vi "CalculateTorque.vi"(4 "Frequency":dbl, 5 "TranslationPosition":dbl, 6 "Sensors Right":T1, 7 "Sensors Left":T1) -> (3 "Torque":dbl)   [LabVIEW 2019]
uses:
  <vilib>/Utility/miscctls.llb/LV3DPointTypeDef.ctl
  <vilib>/Analysis/Matrix/Datatypes/RealMatrix.ctl
  TypeDefs/SensorControl.ctl
  <vilib>/Analysis/3filter.llb/Filter Passband Type.ctl
  <vilib>/Analysis/_algsub.llb/Real Vector Norm.vi
  <vilib>/Analysis/baseanly.llb/A x Vector.vi
  <vilib>/Analysis/NI_AALBase.lvlib
  <vilib>/Analysis/NI_AALPro.lvlib
  <vilib>/ptbypt/NI_PtbyPt.lvlib
  <vilib>/Analysis/Matrix/NI_Matrix.lvlib
panel:
  out "RotMatrix":T2
  out "size right":i32
  out "Vertex Array right":T3[](array[typedef])
  out "triangle":dbl[](array[numeric])
  out "size left":i32
  out "Vertex Array left":T3[](array[typedef])
  out "Low Cutoff":dbl=30.0
  out "t_right":dbl format="%.2f"
  out "intersect_right":bool
  out "t_left":dbl format="%.2f"
  out "intersect_left":bool
  out "dir left":dbl[](array[numeric])
  out "orig left":dbl[](array[numeric])
  out "dir right":dbl[](array[numeric])
  out "orig right":dbl[](array[numeric])
  out "force left":dbl[](array[numeric])
  out "force right":dbl[](array[numeric])
  out "torque left":dbl[](array[numeric])
  out "torque right":dbl[](array[numeric])
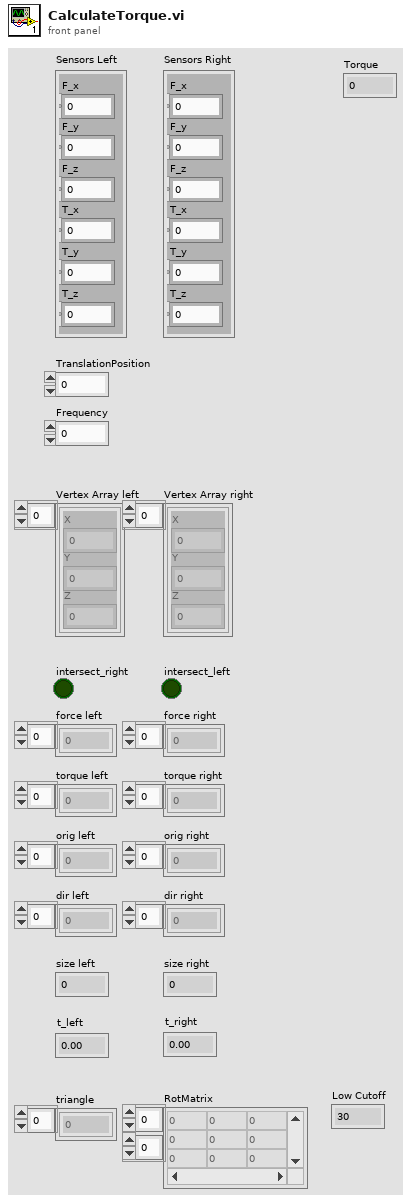
[diagram p1: front panel]
types:
  T1 = typedef "SensorControl.ctl" = cluster{"F_x":dbl, "F_y":dbl, "F_z":dbl, "T_x":dbl, "T_y":dbl, "T_z":dbl}
  T2 = typedef "NI_Matrix.lvlib/RealMatrix.ctl" = dbl[][]
  T3 = typedef "LV3DPointTypeDef.ctl" = cluster{"X":sgl, "Y":sgl, "Z":sgl}
  T4 = typedef "NI_AALBase.lvlib/Filter Passband Type.ctl" = enum32{"Lowpass", "Highpass", "Bandpass", "Bandstop"}
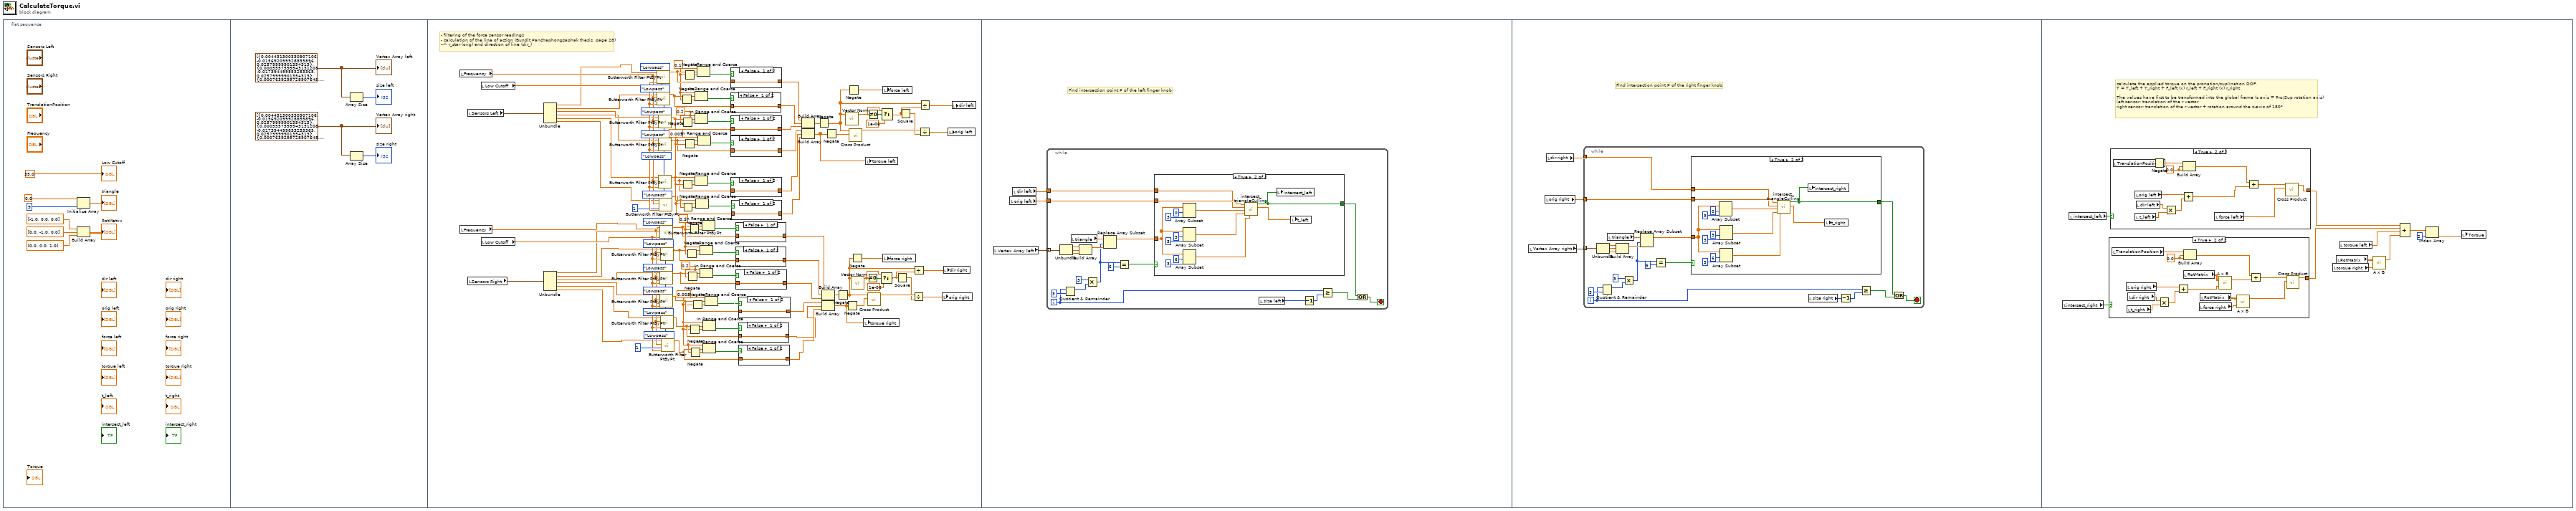
[diagram p0: block diagram]
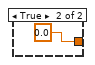
[diagram p2: hidden frame]
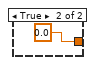
[diagram p3: hidden frame]
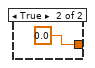
[diagram p4: hidden frame]
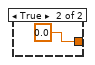
[diagram p5: hidden frame]
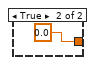
[diagram p6: hidden frame]
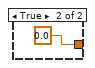
[diagram p7: hidden frame]
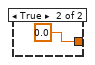
[diagram p8: hidden frame]
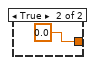
[diagram p9: hidden frame]
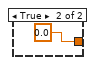
[diagram p10: hidden frame]
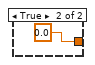
[diagram p11: hidden frame]
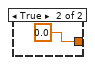
[diagram p12: hidden frame]
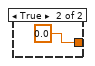
[diagram p13: hidden frame]
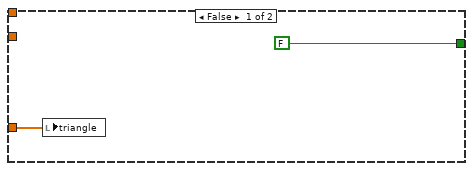
[diagram p14: hidden frame]
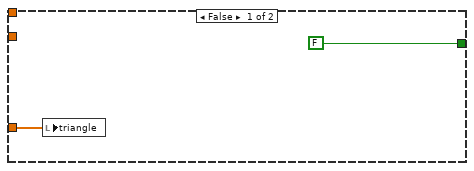
[diagram p15: hidden frame]
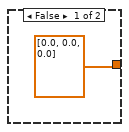
[diagram p16: hidden frame]
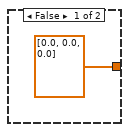
[diagram p17: hidden frame]
diagram:
  n1 = flat-sequence {
    frame #0 {
      n2 = Initialize Array(0.0 ("element"), 9 ("dimension size")) -> (→"triangle":dbl[])
      n3 = Build Array(dbl[] [-1.0, 0.0, 0.0] ("element"), dbl[] [0.0, -1.0, 0.0] ("element"), dbl[] [0.0, 0.0, 1.0] ("element")) -> (→"RotMatrix":T2)
      "Low Cutoff" <- 35.0
    }
    frame #1 {
      w11 = T3[] [{"X"=0.0044313003, "Y"=-0.0156921, "Z"=0.025799999}, {"X"=0.00055576, "Y"=-0.0173945, "Z"=0.025799999}, {"X"=0.00076393, "Y"=-0.02, "Z"=0.025799999}, {"X"=0.00076393, "Y"=-0.02, "Z"=0.025799999}, {"X"=0.00076393, "Y"=-0.02, "Z"=0.0088}, {"X"=0.00055576, "Y"=-0.0173945, "Z"=0.0088}, {"X"=0.00044313, "Y"=-0.0156921, "Z"=0.025799999}, {"X"=0.00055576, "Y"=-0.0173945, "Z"=0.0088}, {"X"=0.00044313, "Y"=-0.0156921, "Z"=0.0088}, {"X"=0.00044313, "Y"=-0.0156921, "Z"=0.025799999}, {"X"=0.00076393, "Y"=-0.02, "Z"=0.025799999}, {"X"=0.00055576, "Y"=-0.0173945, "Z"=0.0088}, {"X"=0.00044313, "Y"=-0.0156921, "Z"=0.0088}, {"X"=0.0002803, "Y"=-0.012661899, "Z"=0.0088}, {"X"=0.0002803, "Y"=-0.012661899, "Z"=0.025799999}, {"X"=0.0002803, "Y"=-0.012661899, "Z"=0.025799999}, {"X"=0.00044313, "Y"=-0.0156921, "Z"=0.025799999}, {"X"=0.00044313, "Y"=-0.0156921, "Z"=0.0088}, {"X"=0.00026629, "Y"=-0.0120288, "Z"=0.025799999}, {"X"=0.00026629, "Y"=-0.0120288, "Z"=0.0088}, {"X"=0.00028451, "Y"=-0.0113124, "Z"=0.0088}, {"X"=0.00030813, "Y"=-0.0109895, "Z"=0.0088}, {"X"=0.00033954, "Y"=-0.01074, "Z"=0.0088}, {"X"=0.00033954, "Y"=-0.01074, "Z"=0.025799999}, {"X"=0.00033954, "Y"=-0.01074, "Z"=0.025799999}, {"X"=0.00026629, "Y"=-0.0120288, "Z"=0.025799999}, {"X"=0.00028451, "Y"=-0.0113124, "Z"=0.0088}, {"X"=0.00028451, "Y"=-0.0113124, "Z"=0.0088}, {"X"=0.00030813, "Y"=-0.0109895, "Z"=0.0088}, {"X"=0.00033954, "Y"=-0.01074, "Z"=0.025799999}, {"X"=0.00026629, "Y"=-0.0120288, "Z"=0.0088}, {"X"=0.00026629, "Y"=-0.0120288, "Z"=0.025799999}, {"X"=0.0002803, "Y"=-0.012661899, "Z"=0.025799999}, {"X"=0.0002803, "Y"=-0.012661899, "Z"=0.025799999}, {"X"=0.0002803, "Y"=-0.012661899, "Z"=0.0088}, {"X"=0.00026629, "Y"=-0.0120288, "Z"=0.0088}, {"X"=0.00044204, "Y"=-0.0100592, "Z"=0.025799999}, {"X"=0.00033954, "Y"=-0.01074, "Z"=0.025799999}, {"X"=0.00033954, "Y"=-0.01074, "Z"=0.0088}, {"X"=0.00033954, "Y"=-0.01074, "Z"=0.0088}, {"X"=0.00079033, "Y"=-0.0061129997, "Z"=0.0088}, {"X"=0.00079033, "Y"=-0.0061129997, "Z"=0.025799999}, {"X"=0.00079033, "Y"=-0.0061129997, "Z"=0.025799999}, {"X"=0.00044204, "Y"=-0.0100592, "Z"=0.025799999}, {"X"=0.00033954, "Y"=-0.01074, "Z"=0.0088}, {"X"=0.00094135, "Y"=-0.0014677, "Z"=0.025799999}, {"X"=0.00079033, "Y"=-0.0061129997, "Z"=0.025799999}, {"X"=0.00079033, "Y"=-0.0061129997, "Z"=0.0088}, {"X"=0.00079033, "Y"=-0.0061129997, "Z"=0.0088}, {"X"=0.00095, "Y"=0.0, "Z"=0.0088}, {"X"=0.00095, "Y"=0.0, "Z"=0.025799999}, {"X"=0.00095, "Y"=0.0, "Z"=0.025799999}, {"X"=0.00094135, "Y"=-0.0014677, "Z"=0.025799999}, {"X"=0.00079033, "Y"=-0.0061129997, "Z"=0.0088}, {"X"=0.00079033, "Y"=0.0061129997, "Z"=0.025799999}, {"X"=0.00095, "Y"=0.0, "Z"=0.025799999}, {"X"=0.00095, "Y"=0.0, "Z"=0.0088}, {"X"=0.00095, "Y"=0.0, "Z"=0.0088}, {"X"=0.00079033, "Y"=0.0061129997, "Z"=0.0088}, {"X"=0.00079033, "Y"=0.0061129997, "Z"=0.025799999}, {"X"=0.00079033, "Y"=0.0061129997, "Z"=0.0088}, {"X"=0.00053803, "Y"=0.0092747, "Z"=0.0088}, {"X"=0.00033954, "Y"=0.01074, "Z"=0.0088}, {"X"=0.00033954, "Y"=0.01074, "Z"=0.0088}, {"X"=0.00033954, "Y"=0.01074, "Z"=0.025799999}, {"X"=0.00067254, "Y"=0.007852701, "Z"=0.025799999}, {"X"=0.00067254, "Y"=0.007852701, "Z"=0.025799999}, {"X"=0.00079033, "Y"=0.0061129997, "Z"=0.025799999}, {"X"=0.00079033, "Y"=0.0061129997, "Z"=0.0088}, {"X"=0.00079033, "Y"=0.0061129997, "Z"=0.0088}, {"X"=0.00033954, "Y"=0.01074, "Z"=0.0088}, {"X"=0.00067254, "Y"=0.007852701, "Z"=0.025799999}, {"X"=0.00026629, "Y"=0.0120289, "Z"=0.025799999}, {"X"=0.00026629, "Y"=0.0120289, "Z"=0.0088}, {"X"=0.0002803, "Y"=0.012661899, "Z"=0.0088}, {"X"=0.0002803, "Y"=0.012661899, "Z"=0.0088}, {"X"=0.0002803, "Y"=0.012661899, "Z"=0.025799999}, {"X"=0.00026629, "Y"=0.0120289, "Z"=0.025799999}, {"X"=0.00026629, "Y"=0.0120289, "Z"=0.0088}, {"X"=0.00026629, "Y"=0.0120289, "Z"=0.025799999}, {"X"=0.0002845, "Y"=0.0113124, "Z"=0.025799999}, {"X"=0.00030813, "Y"=0.0109895, "Z"=0.025799999}, {"X"=0.00033954, "Y"=0.01074, "Z"=0.025799999}, {"X"=0.00033954, "Y"=0.01074, "Z"=0.0088}, {"X"=0.00033954, "Y"=0.01074, "Z"=0.0088}, {"X"=0.00026629, "Y"=0.0120289, "Z"=0.0088}, {"X"=0.0002845, "Y"=0.0113124, "Z"=0.025799999}, {"X"=0.0002845, "Y"=0.0113124, "Z"=0.025799999}, {"X"=0.00030813, "Y"=0.0109895, "Z"=0.025799999}, {"X"=0.00033954, "Y"=0.01074, "Z"=0.0088}, {"X"=0.00044313, "Y"=0.0156921, "Z"=0.025799999}, {"X"=0.0002803, "Y"=0.012661899, "Z"=0.025799999}, {"X"=0.0002803, "Y"=0.012661899, "Z"=0.0088}, {"X"=0.0002803, "Y"=0.012661899, "Z"=0.0088}, {"X"=0.00044313, "Y"=0.0156921, "Z"=0.0088}, {"X"=0.00044313, "Y"=0.0156921, "Z"=0.025799999}, {"X"=0.00062176, "Y"=0.0182866, "Z"=0.0088}, {"X"=0.00076393, "Y"=0.02, "Z"=0.0088}, {"X"=0.00076393, "Y"=0.02, "Z"=0.025799999}, {"X"=0.00055576, "Y"=0.0173945, "Z"=0.025799999}, {"X"=0.00044313, "Y"=0.0156921, "Z"=0.025799999}, {"X"=0.00044313, "Y"=0.0156921, "Z"=0.0088}, {"X"=0.00044313, "Y"=0.0156921, "Z"=0.0088}, {"X"=0.00062176, "Y"=0.0182866, "Z"=0.0088}, {"X"=0.00076393, "Y"=0.02, "Z"=0.025799999}, {"X"=0.00076393, "Y"=0.02, "Z"=0.025799999}, {"X"=0.00055576, "Y"=0.0173945, "Z"=0.025799999}, {"X"=0.00044313, "Y"=0.0156921, "Z"=0.0088}] ("Vertex Array left")
      w10 = T3[] [{"X"=0.0044313003, "Y"=-0.0156921, "Z"=0.025799999}, {"X"=0.00055576, "Y"=-0.0173945, "Z"=0.025799999}, {"X"=0.00076393, "Y"=-0.02, "Z"=0.025799999}, {"X"=0.00076393, "Y"=-0.02, "Z"=0.025799999}, {"X"=0.00076393, "Y"=-0.02, "Z"=0.0088}, {"X"=0.00055576, "Y"=-0.0173945, "Z"=0.0088}, {"X"=0.00044313, "Y"=-0.0156921, "Z"=0.025799999}, {"X"=0.00055576, "Y"=-0.0173945, "Z"=0.0088}, {"X"=0.00044313, "Y"=-0.0156921, "Z"=0.0088}, {"X"=0.00044313, "Y"=-0.0156921, "Z"=0.025799999}, {"X"=0.00076393, "Y"=-0.02, "Z"=0.025799999}, {"X"=0.00055576, "Y"=-0.0173945, "Z"=0.0088}, {"X"=0.00044313, "Y"=-0.0156921, "Z"=0.0088}, {"X"=0.0002803, "Y"=-0.012661899, "Z"=0.0088}, {"X"=0.0002803, "Y"=-0.012661899, "Z"=0.025799999}, {"X"=0.0002803, "Y"=-0.012661899, "Z"=0.025799999}, {"X"=0.00044313, "Y"=-0.0156921, "Z"=0.025799999}, {"X"=0.00044313, "Y"=-0.0156921, "Z"=0.0088}, {"X"=0.00026629, "Y"=-0.0120288, "Z"=0.025799999}, {"X"=0.00026629, "Y"=-0.0120288, "Z"=0.0088}, {"X"=0.00028451, "Y"=-0.0113124, "Z"=0.0088}, {"X"=0.00030813, "Y"=-0.0109895, "Z"=0.0088}, {"X"=0.00033954, "Y"=-0.01074, "Z"=0.0088}, {"X"=0.00033954, "Y"=-0.01074, "Z"=0.025799999}, {"X"=0.00033954, "Y"=-0.01074, "Z"=0.025799999}, {"X"=0.00026629, "Y"=-0.0120288, "Z"=0.025799999}, {"X"=0.00028451, "Y"=-0.0113124, "Z"=0.0088}, {"X"=0.00028451, "Y"=-0.0113124, "Z"=0.0088}, {"X"=0.00030813, "Y"=-0.0109895, "Z"=0.0088}, {"X"=0.00033954, "Y"=-0.01074, "Z"=0.025799999}, {"X"=0.00026629, "Y"=-0.0120288, "Z"=0.0088}, {"X"=0.00026629, "Y"=-0.0120288, "Z"=0.025799999}, {"X"=0.0002803, "Y"=-0.012661899, "Z"=0.025799999}, {"X"=0.0002803, "Y"=-0.012661899, "Z"=0.025799999}, {"X"=0.0002803, "Y"=-0.012661899, "Z"=0.0088}, {"X"=0.00026629, "Y"=-0.0120288, "Z"=0.0088}, {"X"=0.00044204, "Y"=-0.0100592, "Z"=0.025799999}, {"X"=0.00033954, "Y"=-0.01074, "Z"=0.025799999}, {"X"=0.00033954, "Y"=-0.01074, "Z"=0.0088}, {"X"=0.00033954, "Y"=-0.01074, "Z"=0.0088}, {"X"=0.00079033, "Y"=-0.0061129997, "Z"=0.0088}, {"X"=0.00079033, "Y"=-0.0061129997, "Z"=0.025799999}, {"X"=0.00079033, "Y"=-0.0061129997, "Z"=0.025799999}, {"X"=0.00044204, "Y"=-0.0100592, "Z"=0.025799999}, {"X"=0.00033954, "Y"=-0.01074, "Z"=0.0088}, {"X"=0.00094135, "Y"=-0.0014677, "Z"=0.025799999}, {"X"=0.00079033, "Y"=-0.0061129997, "Z"=0.025799999}, {"X"=0.00079033, "Y"=-0.0061129997, "Z"=0.0088}, {"X"=0.00079033, "Y"=-0.0061129997, "Z"=0.0088}, {"X"=0.00095, "Y"=0.0, "Z"=0.0088}, {"X"=0.00095, "Y"=0.0, "Z"=0.025799999}, {"X"=0.00095, "Y"=0.0, "Z"=0.025799999}, {"X"=0.00094135, "Y"=-0.0014677, "Z"=0.025799999}, {"X"=0.00079033, "Y"=-0.0061129997, "Z"=0.0088}, {"X"=0.00079033, "Y"=0.0061129997, "Z"=0.025799999}, {"X"=0.00095, "Y"=0.0, "Z"=0.025799999}, {"X"=0.00095, "Y"=0.0, "Z"=0.0088}, {"X"=0.00095, "Y"=0.0, "Z"=0.0088}, {"X"=0.00079033, "Y"=0.0061129997, "Z"=0.0088}, {"X"=0.00079033, "Y"=0.0061129997, "Z"=0.025799999}, {"X"=0.00079033, "Y"=0.0061129997, "Z"=0.0088}, {"X"=0.00053803, "Y"=0.0092747, "Z"=0.0088}, {"X"=0.00033954, "Y"=0.01074, "Z"=0.0088}, {"X"=0.00033954, "Y"=0.01074, "Z"=0.0088}, {"X"=0.00033954, "Y"=0.01074, "Z"=0.025799999}, {"X"=0.00067254, "Y"=0.007852701, "Z"=0.025799999}, {"X"=0.00067254, "Y"=0.007852701, "Z"=0.025799999}, {"X"=0.00079033, "Y"=0.0061129997, "Z"=0.025799999}, {"X"=0.00079033, "Y"=0.0061129997, "Z"=0.0088}, {"X"=0.00079033, "Y"=0.0061129997, "Z"=0.0088}, {"X"=0.00033954, "Y"=0.01074, "Z"=0.0088}, {"X"=0.00067254, "Y"=0.007852701, "Z"=0.025799999}, {"X"=0.00026629, "Y"=0.0120289, "Z"=0.025799999}, {"X"=0.00026629, "Y"=0.0120289, "Z"=0.0088}, {"X"=0.0002803, "Y"=0.012661899, "Z"=0.0088}, {"X"=0.0002803, "Y"=0.012661899, "Z"=0.0088}, {"X"=0.0002803, "Y"=0.012661899, "Z"=0.025799999}, {"X"=0.00026629, "Y"=0.0120289, "Z"=0.025799999}, {"X"=0.00026629, "Y"=0.0120289, "Z"=0.0088}, {"X"=0.00026629, "Y"=0.0120289, "Z"=0.025799999}, {"X"=0.0002845, "Y"=0.0113124, "Z"=0.025799999}, {"X"=0.00030813, "Y"=0.0109895, "Z"=0.025799999}, {"X"=0.00033954, "Y"=0.01074, "Z"=0.025799999}, {"X"=0.00033954, "Y"=0.01074, "Z"=0.0088}, {"X"=0.00033954, "Y"=0.01074, "Z"=0.0088}, {"X"=0.00026629, "Y"=0.0120289, "Z"=0.0088}, {"X"=0.0002845, "Y"=0.0113124, "Z"=0.025799999}, {"X"=0.0002845, "Y"=0.0113124, "Z"=0.025799999}, {"X"=0.00030813, "Y"=0.0109895, "Z"=0.025799999}, {"X"=0.00033954, "Y"=0.01074, "Z"=0.0088}, {"X"=0.00044313, "Y"=0.0156921, "Z"=0.025799999}, {"X"=0.0002803, "Y"=0.012661899, "Z"=0.025799999}, {"X"=0.0002803, "Y"=0.012661899, "Z"=0.0088}, {"X"=0.0002803, "Y"=0.012661899, "Z"=0.0088}, {"X"=0.00044313, "Y"=0.0156921, "Z"=0.0088}, {"X"=0.00044313, "Y"=0.0156921, "Z"=0.025799999}, {"X"=0.00062176, "Y"=0.0182866, "Z"=0.0088}, {"X"=0.00076393, "Y"=0.02, "Z"=0.0088}, {"X"=0.00076393, "Y"=0.02, "Z"=0.025799999}, {"X"=0.00055576, "Y"=0.0173945, "Z"=0.025799999}, {"X"=0.00044313, "Y"=0.0156921, "Z"=0.025799999}, {"X"=0.00044313, "Y"=0.0156921, "Z"=0.0088}, {"X"=0.00044313, "Y"=0.0156921, "Z"=0.0088}, {"X"=0.00062176, "Y"=0.0182866, "Z"=0.0088}, {"X"=0.00076393, "Y"=0.02, "Z"=0.025799999}, {"X"=0.00076393, "Y"=0.02, "Z"=0.025799999}, {"X"=0.00055576, "Y"=0.0173945, "Z"=0.025799999}, {"X"=0.00044313, "Y"=0.0156921, "Z"=0.0088}] ("Vertex Array right")
      n4 = Array Size(array=w11) -> (size(s)=→"size left":i32)
      n5 = Array Size(array=w10) -> (size(s)=→"size right":i32)
      "Vertex Array left" <- w11
      "Vertex Array right" <- w10
    }
    frame #2 {
      w56 = 0.005 ("upper limit")
      w57 = 0.005 ("upper limit")
      w83 = 0.2 ("upper limit")
      w82 = 0.1 ("upper limit")
      w84 = 0.2 ("upper limit")
      w86 = 0.1 ("upper limit")
      w99 = 1 ("order")
      (unwired) Filter_Passband_Type."Lowpass" ("filter type")
      (unwired) Filter_Passband_Type."Lowpass" ("filter type")
      (unwired) Filter_Passband_Type."Lowpass" ("filter type")
      (unwired) Filter_Passband_Type."Lowpass" ("filter type")
      (unwired) Filter_Passband_Type."Lowpass" ("filter type")
      (unwired) Filter_Passband_Type."Lowpass" ("filter type")
      w100 = 1 ("order")
      (unwired) Filter_Passband_Type."Lowpass" ("filter type")
      (unwired) Filter_Passband_Type."Lowpass" ("filter type")
      (unwired) Filter_Passband_Type."Lowpass" ("filter type")
      (unwired) Filter_Passband_Type."Lowpass" ("filter type")
      (unwired) Filter_Passband_Type."Lowpass" ("filter type")
      (unwired) Filter_Passband_Type."Lowpass" ("filter type")
      # "- filtering of the force sensor readings\n- calculation of the line of action (Bundit Panchaphongsaphak thesis, page 28)\n--> r_star (orig) and direction of line (dir_)"
      n6 = local read "Frequency"() -> (w102:dbl)
      n7 = local read "Frequency"() -> (w98:dbl)
      n8 = local read "Sensors Left"() -> (w34:T1)
      n9 = local read "Sensors Right"() -> (w27:T1)
      n10 = local read "Low Cutoff"() -> (w101:dbl)
      n11 = local read "Low Cutoff"() -> (w97:dbl)
      n12 = Unbundle(w34) -> ("F_x"=w33:dbl, "F_y"=w32:dbl, "F_z"=w31:dbl, "T_x"=w30:dbl, "T_y"=w29:dbl, "T_z"=w28:dbl)
      n13 = Unbundle(w27) -> ("F_x"=w26:dbl, "F_y"=w25:dbl, "F_z"=w24:dbl, "T_x"=w23:dbl, "T_y"=w22:dbl, "T_z"=w21:dbl)
      n14 = call <vilib>:"Butterworth Filter PtByPt.vi"("order"=w100, "low cutoff freq: fl"=w101, "sampling freq: fs"=w102, "x"=w33) -> ("Filtered x"=w94:dbl)  [unwired: 5 in, 1 out]
      n15 = call <vilib>:"Butterworth Filter PtByPt.vi"("order"=w100, "low cutoff freq: fl"=w101, "sampling freq: fs"=w102, "x"=w32) -> ("Filtered x"=w91:dbl)  [unwired: 5 in, 1 out]
      n16 = call <vilib>:"Butterworth Filter PtByPt.vi"("order"=w100, "low cutoff freq: fl"=w101, "sampling freq: fs"=w102, "x"=w31) -> ("Filtered x"=w87:dbl)  [unwired: 5 in, 1 out]
      n17 = call <vilib>:"Butterworth Filter PtByPt.vi"("order"=w100, "low cutoff freq: fl"=w101, "sampling freq: fs"=w102, "x"=w30) -> ("Filtered x"=w49:dbl)  [unwired: 5 in, 1 out]
      n18 = call <vilib>:"Butterworth Filter PtByPt.vi"("order"=w100, "low cutoff freq: fl"=w101, "sampling freq: fs"=w102, "x"=w29) -> ("Filtered x"=w48:dbl)  [unwired: 5 in, 1 out]
      n19 = call <vilib>:"Butterworth Filter PtByPt.vi"("order"=w100, "low cutoff freq: fl"=w101, "sampling freq: fs"=w102, "x"=w28) -> ("Filtered x"=w47:dbl)  [unwired: 5 in, 1 out]
      n20 = call <vilib>:"Butterworth Filter PtByPt.vi"("order"=w99, "low cutoff freq: fl"=w97, "sampling freq: fs"=w98, "x"=w26) -> ("Filtered x"=w75:dbl)  [unwired: 5 in, 1 out]
      n21 = call <vilib>:"Butterworth Filter PtByPt.vi"("order"=w99, "low cutoff freq: fl"=w97, "sampling freq: fs"=w98, "x"=w24) -> ("Filtered x"=w74:dbl)  [unwired: 5 in, 1 out]
      n22 = call <vilib>:"Butterworth Filter PtByPt.vi"("order"=w99, "low cutoff freq: fl"=w97, "sampling freq: fs"=w98, "x"=w23) -> ("Filtered x"=w63:dbl)  [unwired: 5 in, 1 out]
      n23 = call <vilib>:"Butterworth Filter PtByPt.vi"("order"=w99, "low cutoff freq: fl"=w97, "sampling freq: fs"=w98, "x"=w25) -> ("Filtered x"=w70:dbl)  [unwired: 5 in, 1 out]
      n24 = call <vilib>:"Butterworth Filter PtByPt.vi"("order"=w99, "low cutoff freq: fl"=w97, "sampling freq: fs"=w98, "x"=w22) -> ("Filtered x"=w62:dbl)  [unwired: 5 in, 1 out]
      n25 = call <vilib>:"Butterworth Filter PtByPt.vi"("order"=w99, "low cutoff freq: fl"=w97, "sampling freq: fs"=w98, "x"=w21) -> ("Filtered x"=w61:dbl)  [unwired: 5 in, 1 out]
      n26 = Negate(x=w86) -> (-x=w92:dbl)
      n27 = Negate(x=w84) -> (-x=w89:dbl)
      n28 = Negate(x=w56) -> (-x=w53:dbl)
      n29 = Negate(x=w56) -> (-x=w54:dbl)
      n30 = Negate(x=w86) -> (-x=w96:dbl)
      n31 = Negate(x=w56) -> (-x=w50:dbl)
      n32 = Negate(x=w82) -> (-x=w79:dbl)
      n33 = Negate(x=w83) -> (-x=w80:dbl)
      n34 = Negate(x=w82) -> (-x=w76:dbl)
      n35 = Negate(x=w57) -> (-x=w66:dbl)
      n36 = Negate(x=w57) -> (-x=w65:dbl)
      n37 = Negate(x=w57) -> (-x=w69:dbl)
      n38 = In Range and Coerce(upper limit=w86, x=w91, lower limit=w92) -> (In Range?=w93:bool)  [unwired: 1 out]
      n39 = In Range and Coerce(upper limit=w84, x=w87, lower limit=w89) -> (In Range?=w88:bool)  [unwired: 1 out]
      n40 = In Range and Coerce(upper limit=w56, x=w48, lower limit=w53) -> (In Range?=w52:bool)  [unwired: 1 out]
      n41 = In Range and Coerce(upper limit=w56, x=w47, lower limit=w54) -> (In Range?=w55:bool)  [unwired: 1 out]
      n42 = In Range and Coerce(upper limit=w86, x=w94, lower limit=w96) -> (In Range?=w95:bool)  [unwired: 1 out]
      n43 = In Range and Coerce(upper limit=w56, x=w49, lower limit=w50) -> (In Range?=w51:bool)  [unwired: 1 out]
      n44 = In Range and Coerce(upper limit=w82, x=w70, lower limit=w79) -> (In Range?=w78:bool)  [unwired: 1 out]
      n45 = In Range and Coerce(upper limit=w83, x=w74, lower limit=w80) -> (In Range?=w81:bool)  [unwired: 1 out]
      n46 = In Range and Coerce(upper limit=w82, x=w75, lower limit=w76) -> (In Range?=w77:bool)  [unwired: 1 out]
      n47 = In Range and Coerce(upper limit=w57, x=w62, lower limit=w66) -> (In Range?=w67:bool)  [unwired: 1 out]
      n48 = In Range and Coerce(upper limit=w57, x=w61, lower limit=w65) -> (In Range?=w64:bool)  [unwired: 1 out]
      n49 = In Range and Coerce(upper limit=w57, x=w63, lower limit=w69) -> (In Range?=w68:bool)  [unwired: 1 out]
      n50 = case shown="False" w93 {
        tunnel: w91 -> [w133 _]
        tunnel: [w133 0.0 ("element")] -> w90
        frame False {
        }
        frame True {
        }
      }
      n51 = case shown="False" w95 {
        tunnel: w94 -> [w135 _]
        tunnel: [w135 0.0 ("element")] -> w35
        frame False {
        }
        frame True {
        }
      }
      n52 = case shown="False" w88 {
        tunnel: w87 -> [w131 _]
        tunnel: [w131 0.0 ("element")] -> w85
        frame False {
        }
        frame True {
        }
      }
      n53 = case shown="False" w51 {
        tunnel: w49 -> [w117 _]
        tunnel: [w117 0.0 ("element")] -> w44
        frame False {
        }
        frame True {
        }
      }
      n54 = case shown="False" w52 {
        tunnel: w48 -> [w115 _]
        tunnel: [w115 0.0 ("element")] -> w45
        frame False {
        }
        frame True {
        }
      }
      n55 = case shown="False" w55 {
        tunnel: w47 -> [w113 _]
        tunnel: [w113 0.0 ("element")] -> w46
        frame False {
        }
        frame True {
        }
      }
      n56 = case shown="False" w77 {
        tunnel: w75 -> [w129 _]
        tunnel: [w129 0.0 ("element")] -> w72
        frame False {
        }
        frame True {
        }
      }
      n57 = case shown="False" w78 {
        tunnel: w70 -> [w127 _]
        tunnel: [w127 0.0 ("element")] -> w73
        frame False {
        }
        frame True {
        }
      }
      n58 = case shown="False" w81 {
        tunnel: w74 -> [w125 _]
        tunnel: [w125 0.0 ("element")] -> w71
        frame False {
        }
        frame True {
        }
      }
      n59 = case shown="False" w68 {
        tunnel: w63 -> [w123 _]
        tunnel: [w123 0.0 ("element")] -> w58
        frame False {
        }
        frame True {
        }
      }
      n60 = case shown="False" w67 {
        tunnel: w62 -> [w121 _]
        tunnel: [w121 0.0 ("element")] -> w59
        frame False {
        }
        frame True {
        }
      }
      n61 = case shown="False" w64 {
        tunnel: w61 -> [w119 _]
        tunnel: [w119 0.0 ("element")] -> w60
        frame False {
        }
        frame True {
        }
      }
      n62 = Build Array(w35, w90, w85) -> (w112:dbl[])
      n63 = Build Array(w44, w45, w46) -> (w17:dbl[])
      n64 = Negate(x=w112) -> (-x=w104:dbl[])
      n65 = Build Array(w72, w73, w71) -> (w107:dbl[])
      n66 = Build Array(w58, w59, w60) -> (w13:dbl[])
      n67 = Negate(x=w17) -> (-x=w103:dbl[])
      n68 = Negate(x=w107) -> (-x=w106:dbl[])
      n69 = call-poly <vilib>:"Vector Norm.vi"("Input Vector"=w104) -> ("norm"=w37:dbl)  [unwired: 9 in, 1 out]
      n70 = Negate(x=w13) -> (-x=w105:dbl[])
      n71 = Negate(x=w104) -> (-x=w20:dbl[])
      n72 = call <vilib>:"Cross Product.vi"("B Vector"=w103, "A Vector"=w104) -> ("Cross Product"=w110:dbl[])  [unwired: 8 in, 1 out]
      n73 = Negate(x=w106) -> (-x=w16:dbl[])
      n74 = call-poly <vilib>:"Vector Norm.vi"("Input Vector"=w106) -> ("norm"=w42:dbl)  [unwired: 9 in, 1 out]
      n75 = local write "torque right"(w13) -> ()
      n76 = local write "torque left"(w17) -> ()
      n77 = Not Equal To 0?(x=w42) -> (x != 0?=w43:bool)
      n78 = Not Equal To 0?(x=w37) -> (x != 0?=w40:bool)
      n79 = call <vilib>:"Cross Product.vi"("B Vector"=w105, "A Vector"=w106) -> ("Cross Product"=w109:dbl[])  [unwired: 8 in, 1 out]
      n80 = Select(t=w42, s=w43, f=1e-06) -> (s? t:f=w41:dbl)
      n81 = Select(t=w37, s=w40, f=1e-06) -> (s? t:f=w36:dbl)
      n82 = local write "force left"(w20) -> ()
      n83 = local write "force right"(w16) -> ()
      n84 = Square(x=w41) -> (x^2=w108:dbl)
      n85 = Square(x=w36) -> (x^2=w111:dbl)
      n86 = Divide(x=w109, y=w108) -> (x/y=w14:dbl[])
      n87 = Divide(x=w106, y=w41) -> (x/y=w15:dbl[])
      n88 = Divide(x=w110, y=w111) -> (x/y=w18:dbl[])
      n89 = Divide(x=w104, y=w36) -> (x/y=w19:dbl[])
      n90 = local write "orig right"(w14) -> ()
      n91 = local write "dir right"(w15) -> ()
      n92 = local write "orig left"(w18) -> ()
      n93 = local write "dir left"(w19) -> ()
    }
    frame #3 {
      # "Find intersection point P of the left finger knob"
      n94 = local read "Vertex Array left"() -> (w137:T3[])
      n95 = local read "orig left"() -> (w138:dbl[])
      n96 = local read "dir left"() -> (w139:dbl[])
      n97 = while {
        tunnel: w137 -> [w160] mode=indexing
        tunnel: w139 -> [w147]
        tunnel: w138 -> [w146]
        i -> [w140]
        stop <- w145 stop-if-true
        n98 = Unbundle(w160) -> ("X"=w157:sgl, "Y"=w156:sgl, "Z"=w155:sgl)
        n99 = Quotient & Remainder(x=w140, y=3) -> (x-y*floor(x/y)=w152:i32)  [unwired: 1 out]
        n100 = local read "triangle"() -> (w159:dbl[])
        n101 = Build Array(w157, w156, w155) -> (w154:sgl[])
        n102 = Multiply(x=3, y=w152) -> (x*y=w151:i32)
        n103 = Replace Array Subset(array=w159, new element=w154, index=w151) -> (w148:dbl[])
        n104 = Equal?(x=w151, y=6) -> (x = y?=w149:bool)
        n105 = case shown="True" w149 {
          tunnel: w148 -> [w162 w170]
          tunnel: w147 -> [_ w168]
          tunnel: w146 -> [_ w169]
          tunnel: [FALSE ("intersect") w164] -> w144
          frame False {
            n106 = local write "triangle"(w162) -> ()
          }
          frame True {
            n107 = Array Subset(array=w170, index=0, length=3) -> (w167:dbl[])
            n108 = Array Subset(array=w170, index=3, length=3) -> (w166:dbl[])
            n109 = Array Subset(array=w170, index=6, length=3) -> (w165:dbl[])
            n110 = call "intersect_triangleCulling.vi"("vert2"=w165, "vert1"=w166, "vert0"=w167, "dir"=w168, "orig"=w169) -> ("t"=w163:dbl, "intersect"=w164:bool)  [unwired: 2 in, 2 out]
            n111 = local write "intersect_left"(w164) -> ()
            n112 = local write "t_left"(w163) -> ()
          }
        }
        n113 = local read "size left"() -> (w143:i32)
        n114 = Decrement(x=w143) -> (x-1=w141:i32)
        n115 = Greater Or Equal?(x=w140, y=w141) -> (x >= y?=w142:bool)
        n116 = Or(x=w144, y=w142) -> (x .or. y?=w145:bool)
      }
    }
    frame #4 {
      # "Find intersection point P of the right finger knob"
      n117 = local read "Vertex Array right"() -> (w177:T3[])
      n118 = local read "orig right"() -> (w178:dbl[])
      n119 = local read "dir right"() -> (w179:dbl[])
      n120 = while {
        tunnel: w177 -> [w200] mode=indexing
        tunnel: w179 -> [w187]
        tunnel: w178 -> [w186]
        i -> [w180]
        stop <- w185 stop-if-true
        n121 = Unbundle(w200) -> ("X"=w197:sgl, "Y"=w196:sgl, "Z"=w195:sgl)
        n122 = Quotient & Remainder(x=w180, y=3) -> (x-y*floor(x/y)=w192:i32)  [unwired: 1 out]
        n123 = local read "triangle"() -> (w199:dbl[])
        n124 = Build Array(w197, w196, w195) -> (w194:sgl[])
        n125 = Multiply(x=3, y=w192) -> (x*y=w191:i32)
        n126 = Replace Array Subset(array=w199, new element=w194, index=w191) -> (w188:dbl[])
        n127 = Equal?(x=w191, y=6) -> (x = y?=w189:bool)
        n128 = case shown="True" w189 {
          tunnel: w188 -> [w202 w210]
          tunnel: w187 -> [_ w208]
          tunnel: w186 -> [_ w209]
          tunnel: [FALSE ("intersect") w204] -> w184
          frame False {
            n129 = local write "triangle"(w202) -> ()
          }
          frame True {
            n130 = Array Subset(array=w210, index=0, length=3) -> (w207:dbl[])
            n131 = Array Subset(array=w210, index=3, length=3) -> (w206:dbl[])
            n132 = Array Subset(array=w210, index=6, length=3) -> (w205:dbl[])
            n133 = call "intersect_triangleCulling.vi"("vert2"=w205, "vert1"=w206, "vert0"=w207, "dir"=w208, "orig"=w209) -> ("t"=w203:dbl, "intersect"=w204:bool)  [unwired: 2 in, 2 out]
            n134 = local write "intersect_right"(w204) -> ()
            n135 = local write "t_right"(w203) -> ()
          }
        }
        n136 = local read "size right"() -> (w183:i32)
        n137 = Decrement(x=w183) -> (x-1=w181:i32)
        n138 = Greater Or Equal?(x=w180, y=w181) -> (x >= y?=w182:bool)
        n139 = Or(x=w184, y=w182) -> (x .or. y?=w185:bool)
      }
    }
    frame #5 {
      # "calculate the applied torque on the pronation/suplination DOF.\nT = T_left + T_right + F_left (x) r_left + F_right (x) r_right\n\nThe values have first to be transformed into the global frame (z axis = Pro/Sup rotation axis)\nleft sensor: translation of the r vector\nright sensor: translation of the r vector + rotation around the z-axis of 180°"
      n140 = local read "intersect_right"() -> (w226:bool)
      n141 = local read "intersect_left"() -> (w227:bool)
      n142 = case shown="True" w226 {
        tunnel: [dbl[] [0.0, 0.0, 0.0] ("Cross Product") w233] -> w224
        frame False {
        }
        frame True {
          w242 = 0.0 ("element")
          n143 = local read "TranslationPosition"() -> (w229:dbl)
          n144 = local read "orig right"() -> (w240:dbl[])
          n145 = local read "t_right"() -> (w239:dbl)
          n146 = local read "dir right"() -> (w238:dbl[])
          n147 = Multiply(x=w238, y=w239) -> (x*y=w241:dbl[])
          n148 = Add(x=w240, y=w241) -> (x+y=w231:dbl[])
          n149 = local read "RotMatrix"() -> (w232:T2)
          n150 = Build Array(w229, w242, w242) -> (w243:dbl[])
          n151 = local read "force right"() -> (w235:dbl[])
          n152 = local read "RotMatrix"() -> (w236:T2)
          n153 = call-poly <vilib>:"A x B.vi"("Vector"=w231, "A"=w232) -> ("A x Vector"=w230:dbl[])  [unwired: 1 out]
          n154 = call-poly <vilib>:"A x B.vi"("Vector"=w235, "A"=w236) -> ("A x Vector"=w234:dbl[])  [unwired: 1 out]
          n155 = Add(x=w243, y=w230) -> (x+y=w237:dbl[])
          n156 = call <vilib>:"Cross Product.vi"("B Vector"=w234, "A Vector"=w237) -> ("Cross Product"=w233:dbl[])  [unwired: 8 in, 1 out]
        }
      }
      n157 = case shown="True" w227 {
        tunnel: [dbl[] [0.0, 0.0, 0.0] ("Cross Product") w248] -> w225
        frame False {
        }
        frame True {
          w251 = 0.0 ("element")
          n158 = local read "TranslationPosition"() -> (w252:dbl)
          n159 = local read "orig left"() -> (w254:dbl[])
          n160 = local read "t_left"() -> (w255:dbl)
          n161 = local read "dir left"() -> (w256:dbl[])
          n162 = Negate(x=w252) -> (-x=w245:dbl)
          n163 = Multiply(x=w256, y=w255) -> (x*y=w253:dbl[])
          n164 = Add(x=w254, y=w253) -> (x+y=w246:dbl[])
          n165 = Build Array(w245, w251, w251) -> (w250:dbl[])
          n166 = local read "force left"() -> (w247:dbl[])
          n167 = Add(x=w250, y=w246) -> (x+y=w249:dbl[])
          n168 = call <vilib>:"Cross Product.vi"("B Vector"=w247, "A Vector"=w249) -> ("Cross Product"=w248:dbl[])  [unwired: 8 in, 1 out]
        }
      }
      n169 = local read "torque right"() -> (w220:dbl[])
      n170 = local read "RotMatrix"() -> (w221:T2)
      n171 = local read "torque left"() -> (w219:dbl[])
      n172 = call-poly <vilib>:"A x B.vi"("Vector"=w220, "A"=w221) -> ("A x Vector"=w218:dbl[])  [unwired: 1 out]
      n173 = Compound Arithmetic op=ADD(w225, w224, w219, w218) -> (w217:dbl[])
      n174 = Index Array(array=w217, index=2) -> (element=w222:dbl)
      n175 = local write "Torque"(w222) -> ()
    }
  }
